vi "Serial Input Output Tap.vi"(0 "serial input channel resources":T7, 1 "reset":bool, 5 "serial output channel resources":T2, 7 "datapath config":T18 {"channel acq config"."first packet data type select mask" format="%.0x"; "channel acq config"."last packet data type select mask" format="%.0x"}) -> (4 "i2c monitor":T1 {"monitor word" format="%.0x"})   [LabVIEW 2020, in "GettingStarted_Acq_Tap_148X_FPGA.lvlib"]
uses:
  GettingStarted_Acq_Tap_148X_FPGA.lvlib
  Types/Serial Input Channel Datapath Configuration.ctl
  <instrlib>/FlexRIO/CSI-2/v2/FPGA/Types/Channel-Based Acquistion Engine Configuration.ctl
  Types/Serial Input Channel Resources.ctl
  <instrlib>/_niInstr/Memory/v1/FPGA/DRAM/niInstr Memory DRAM v1 FPGA.lvclass
  <instrlib>/FlexRIO/CSI-2/v2/FPGA/DRAM Manager/Private/DRAM Manager.ctl
  <instrlib>/FlexRIO/CSI-2/v2/FPGA/DRAM Manager/Private/Common/DRAM Manager Registers.ctl
  <instrlib>/FlexRIO/CSI-2/v2/FPGA/DRAM Manager/Private/Common/Handshake Registers.ctl
  <instrlib>/FlexRIO/CSI-2/v2/FPGA/DRAM Manager/Private/Common/DRAM Manager FIFOs.ctl
  <instrlib>/FlexRIO/CSI-2/v2/FPGA/DRAM Manager/Private/Common/Write Data FIFO Ref.ctl
  <instrlib>/FlexRIO/CSI-2/v2/FPGA/DRAM Manager/Private/Common/Read Request Metadata FIFO Ref.ctl
  <instrlib>/FlexRIO/CSI-2/v2/FPGA/DRAM Manager/Private/Common/Read Data FIFO Ref.ctl
  Types/Serial Input Channel IO.ctl
  Types/Serial Input Channel IO 32b.ctl
  Types/Serial Input Channel IO 64b.ctl
  Common/Types/I2C IO.ctl
  Types/Serial Ouput Channel Resources.ctl
  Common/Types/Serial Output Channel IO.ctl
  Common/Types/Serial Output Channel IO 32b.ctl
  Common/Types/Serial Output Channel IO 64b.ctl
  <instrlib>/FlexRIO/API/FPGA/v1/IO/NI148x/i2c monitor.ctl
  Common/GettingStarted_Common_148X_FPGA.lvlib
  <instrlib>/FlexRIO/CSI-2/v2/FPGA/NI CSI-2 API FPGA v2.lvlib
  <instrlib>/FlexRIO/CSI-2/v2/FPGA/DRAM Manager/DRAM Manager v2.lvlib
  <instrlib>/FlexRIO/API/FPGA/v1/IO/NI148x/FlexRIO 148x FPGA v1.lvlib
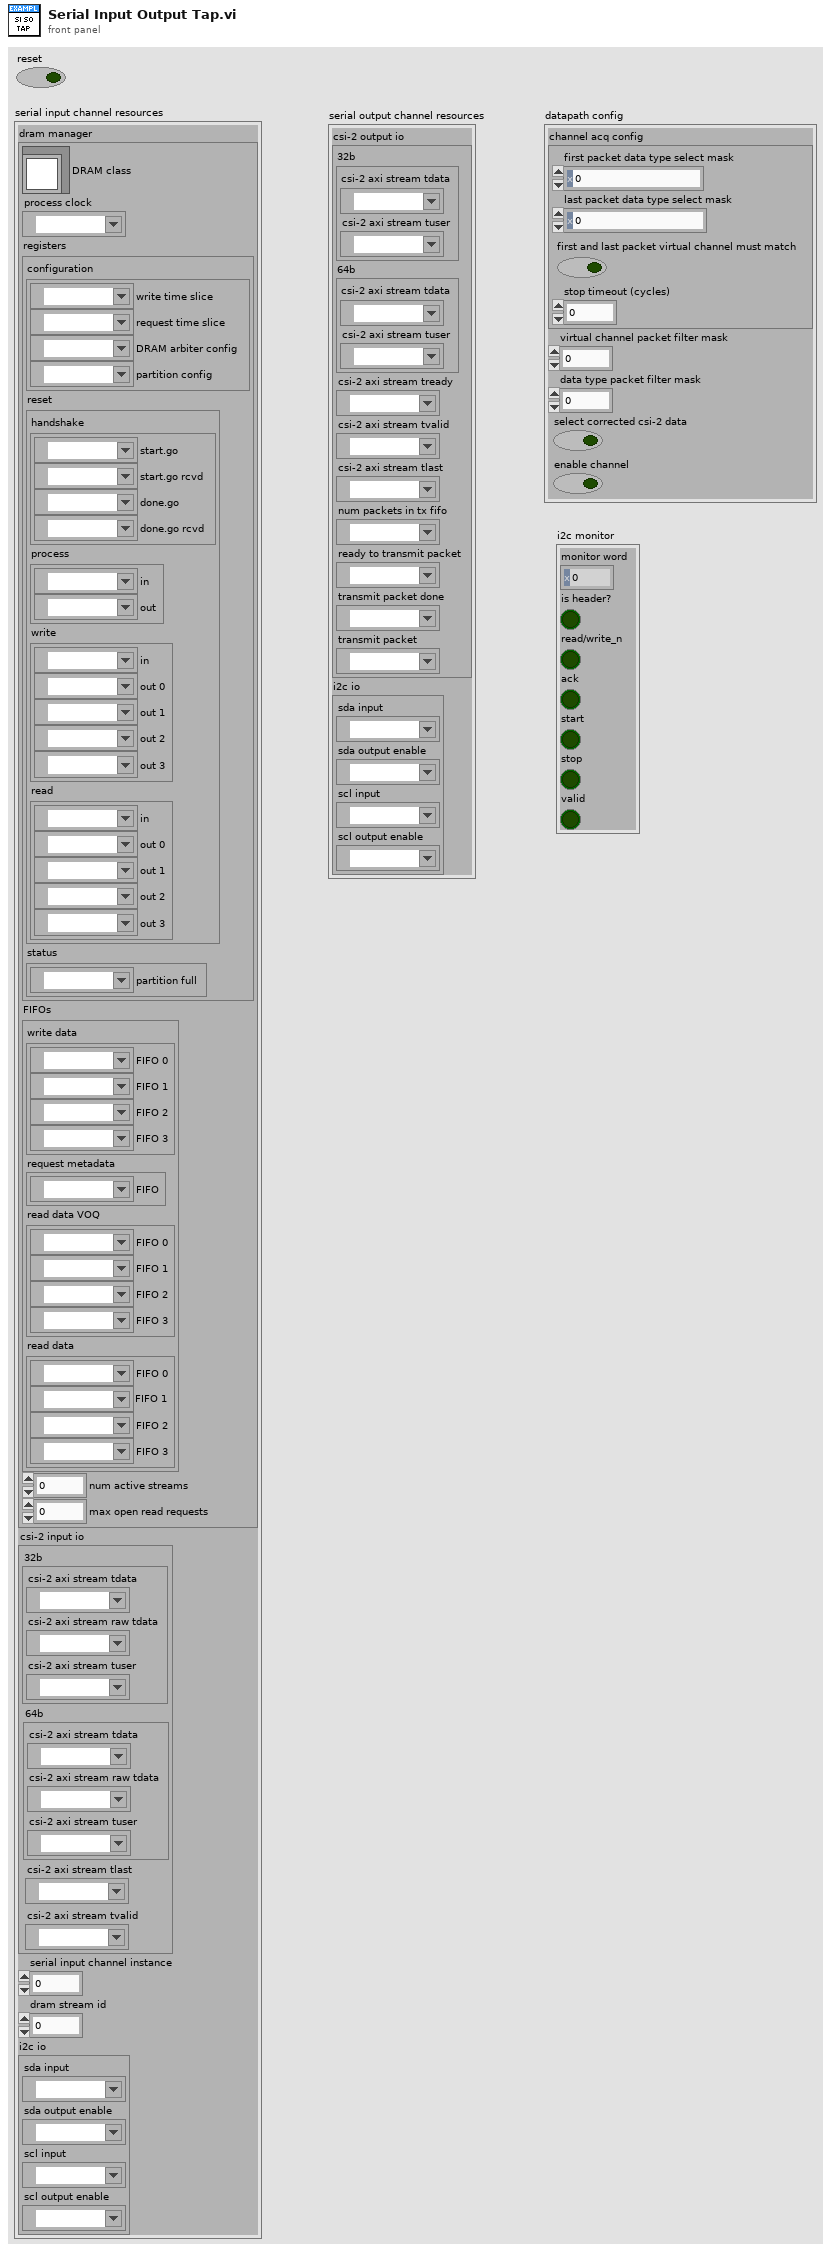
[diagram p1: front panel]
types:
  T1 = typedef "FlexRIO 148x FPGA v1.lvlib/i2c monitor.ctl" = cluster{"monitor word":u8, "is header?":bool, "read/write_n":bool, "ack":bool, "start":bool, "stop":bool, "valid":bool}
  T2 = typedef "GettingStarted_Acq_Tap_148X_FPGA.lvlib/Serial Ouput Channel Resources.ctl" = cluster{"csi-2 output io":T3, "i2c io":T6}
  T3 = typedef "GettingStarted_Common_148X_FPGA.lvlib/Serial Output Channel IO.ctl" = cluster{"32b":T4, "64b":T5, "csi-2 axi stream tready":refnum<k21>, "csi-2 axi stream tvalid":refnum<k21>, "csi-2 axi stream tlast":refnum<k21>, "num packets in tx fifo":refnum<k21>, "ready to transmit packet":refnum<k21>, "transmit packet done":refnum<k21>, "transmit packet":refnum<k21>}
  T4 = typedef "GettingStarted_Common_148X_FPGA.lvlib/Serial Output Channel IO 32b.ctl" = cluster{"csi-2 axi stream tdata":refnum<k21>, "csi-2 axi stream tuser":refnum<k21>}
  T5 = typedef "GettingStarted_Common_148X_FPGA.lvlib/Serial Output Channel IO 64b.ctl" = cluster{"csi-2 axi stream tdata":refnum<k21>, "csi-2 axi stream tuser":refnum<k21>}
  T6 = typedef "GettingStarted_Common_148X_FPGA.lvlib/I2C IO.ctl" = cluster{"sda input":refnum<k21>, "sda output enable":refnum<k21>, "scl input":refnum<k21>, "scl output enable":refnum<k21>}
  T7 = typedef "GettingStarted_Acq_Tap_148X_FPGA.lvlib/Serial Input Channel Resources.ctl" = cluster{"dram manager":T8, "csi-2 input io":T15, "serial input channel instance":u8, "dram stream id":fxp<+,2,2>, "i2c io":T6}
  T8 = typedef "DRAM Manager v2.lvlib/DRAM Manager.ctl" = cluster{"DRAM class":refnum<class "niInstr Memory DRAM v1 FPGA.lvclass">, "process clock":refnum<k21>, "registers":T9, "FIFOs":T11, "num active streams":fxp<+,3,3>, "max open read requests":u16}
  T9 = typedef "DRAM Manager v2.lvlib/DRAM Manager Registers.ctl" = cluster{"configuration":cluster{"write time slice":refnum<k21>, "request time slice":refnum<k21>, "DRAM arbiter config":refnum<k21>, "partition config":refnum<k21>}, "reset":cluster{"handshake":T10, "process":cluster{"in":refnum<k21>, "out":refnum<k21>}, "write":cluster{"in":refnum<k21>, "out 0":refnum<k21>, "out 1":refnum<k21>, "out 2":refnum<k21>, "out 3":refnum<k21>}, "read":cluster{"in":refnum<k21>, "out 0":refnum<k21>, "out 1":refnum<k21>, "out 2":refnum<k21>, "out 3":refnum<k21>}}, "status":cluster{"partition full":refnum<k21>}}
  T10 = typedef "DRAM Manager v2.lvlib/Handshake Registers.ctl" = cluster{"start.go":refnum<k21>, "start.go rcvd":refnum<k21>, "done.go":refnum<k21>, "done.go rcvd":refnum<k21>}
  T11 = typedef "DRAM Manager v2.lvlib/DRAM Manager FIFOs.ctl" = cluster{"write data":cluster{"FIFO 0":T12, "FIFO 1":T12, "FIFO 2":T12, "FIFO 3":T12}, "request metadata":cluster{"FIFO":T13}, "read data VOQ":cluster{"FIFO 0":T14, "FIFO 1":T14, "FIFO 2":T14, "FIFO 3":T14}, "read data":cluster{"FIFO 0":T14, "FIFO 1":T14, "FIFO 2":T14, "FIFO 3":T14}}
  T12 = typedef "DRAM Manager v2.lvlib/Write Data FIFO Ref.ctl" = refnum<k21>
  T13 = typedef "DRAM Manager v2.lvlib/Read Request Metadata FIFO Ref.ctl" = refnum<k21>
  T14 = typedef "DRAM Manager v2.lvlib/Read Data FIFO Ref.ctl" = refnum<k21>
  T15 = typedef "GettingStarted_Acq_Tap_148X_FPGA.lvlib/Serial Input Channel IO.ctl" = cluster{"32b":T16, "64b":T17, "csi-2 axi stream tlast":refnum<k21>, "csi-2 axi stream tvalid":refnum<k21>}
  T16 = typedef "GettingStarted_Acq_Tap_148X_FPGA.lvlib/Serial Input Channel IO 32b.ctl" = cluster{"csi-2 axi stream tdata":refnum<k21>, "csi-2 axi stream raw tdata":refnum<k21>, "csi-2 axi stream tuser":refnum<k21>}
  T17 = typedef "GettingStarted_Acq_Tap_148X_FPGA.lvlib/Serial Input Channel IO 64b.ctl" = cluster{"csi-2 axi stream tdata":refnum<k21>, "csi-2 axi stream raw tdata":refnum<k21>, "csi-2 axi stream tuser":refnum<k21>}
  T18 = typedef "GettingStarted_Acq_Tap_148X_FPGA.lvlib/Serial Input Channel Datapath Configuration.ctl" = cluster{"channel acq config":T19, "virtual channel packet filter mask":u16, "data type packet filter mask":u64, "select corrected csi-2 data":bool, "enable channel":bool}
  T19 = typedef "NI CSI-2 API FPGA v2.lvlib/Channel-Based Acquistion Engine Configuration.ctl" = cluster{"stop timeout (cycles)":u32, "first packet data type select mask":u64, "last packet data type select mask":u64, "first and last packet virtual channel must match":bool}
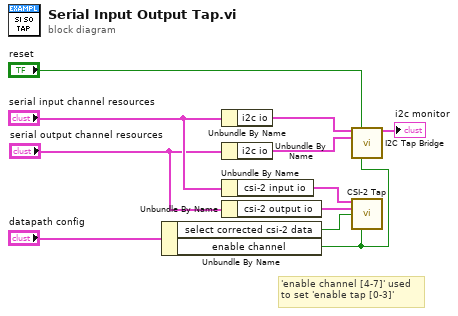
[diagram p0: block diagram]
diagram:
  # "'enable channel [4-7]' used\nto set 'enable tap [0-3]'"
  n1 = Unbundle By Name("datapath config") -> ("select corrected csi-2 data"=w3:bool, "enable channel"=w1:bool)
  n2 = Unbundle By Name("serial input channel resources") -> ("i2c io"=w9:T6)
  n3 = Unbundle By Name("serial output channel resources") -> ("i2c io"=w8:T6)
  n4 = Unbundle By Name("serial input channel resources") -> ("csi-2 input io"=w5:T15)
  n5 = Unbundle By Name("serial output channel resources") -> ("csi-2 output io"=w4:T3)
  n6 = call "I2C Tap Bridge.vi"("input channel i2c io"=w9, "reset"="reset", "output channel i2c io"=w8, "enable i2c tap bridge"=w1) -> ("i2c monitor"=→"i2c monitor":T1)  [unwired: 11 in]
  n7 = call "CSI-2 Tap.vi"("csi-2 input io"=w5, "csi-2 output io"=w4, "select corrected csi-2 data"=w3, "enable tap"=w1) -> ()  [unwired: 11 in, 1 out]
